vi "Using Timestamp and Elapsed Time Functions.vi"() -> ()   [LabVIEW 2019]
panel:
  out "Current Time":timestamp format="%<%x %.3X>T"
  out "Target Time Has Elapsed":bool
  out "Elapsed Time (s)":dbl
  in  "Time Target (s)":dbl=1.0
  in  "Slope (m)":dbl
  in  "x":dbl
  in  "Y-Intercept (b)":dbl
  out "y":dbl
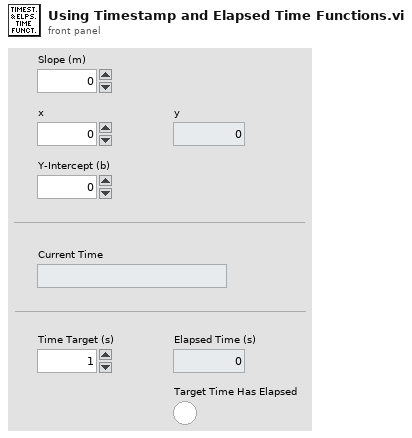
[diagram p1: front panel]
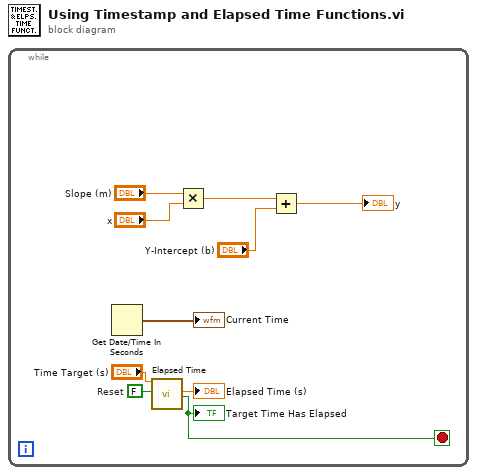
[diagram p0: block diagram]
diagram:
  n1 = while {
    stop <- w2 stop-if-true
    w5 = FALSE  # Reset
    n2 = Get Date/Time In Seconds() -> (seconds since 1Jan1904=→"Current Time":timestamp)
    n3 = call "Elapsed Time"("Time Target (s)"="Time Target (s)", "Reset"=w5) -> ("Elapsed Time (s)"=→"Elapsed Time (s)":dbl, "Time has Elapsed"=w2:bool)  [unwired: 10 in, 6 out]
    "Target Time Has Elapsed" <- w2
    n4 = Multiply(x="Slope (m)", y="x") -> (x*y=w8:dbl)
    n5 = Add(x=w8, y="Y-Intercept (b)") -> (x+y=→"y":dbl)
  }
